vi "fft_kf_update.vi"(9 "Measurement":cdb[](array[numeric]) format="%#_3p", 10 "Measure noise RMS":dbl[](array[numeric]) format="%#_3e", 11 "KF in":T7 {"K" format="%#_2g"; "y lim" format="%#_3g"; "x lim" format="%#_2g"; "P" format="%#_2g"; "H" format="%#_3g"; "x" format="%#_3g"; "Q" format="%#_2g"; "R" format="%#_2g"; "B" format="%#_2g"; "A" format="%#_3g"}) -> (2 "KF out":T7 {"K" format="%#_2g"; "y lim" format="%#_3g"; "x lim" format="%#_2g"; "P" format="%#_2g"; "H" format="%#_3g"; "x" format="%#_3g"; "Q" format="%#_2g"; "R" format="%#_2g"; "B" format="%#_2g"; "A" format="%#_3g"}, 3 "KF estimate":cdb[](array[numeric]) format="%#_3f")   [LabVIEW 2026]
uses:
  utilities/kalman_filter.ctl
  <vilib>/Analysis/Matrix/Datatypes/RealMatrix.ctl
  ilemt_config.ctl
  system/IO_params.ctl
  stft_params.ctl
  <vilib>/Analysis/4window.llb/windowTd.ctl
  filter_params.ctl
  detrend_mode.ctl
  <vilib>/Analysis/Matrix/Numeric/Conversions/Array To Matrix - RA2.vi
  <vilib>/Analysis/Matrix/NI_Matrix.lvlib
  <vilib>/Analysis/NI_AALPro.lvlib
panel:
  in  "Config":T1={"IO params"={"Conversion"={"Rate"=4.0, "Num cards"=2, "Out channels"=4}, "Carriers"={"Phase shift"=180.0, "Levels"=[[0.8, 0.8, 0.8], [0.03, 0.03, 0.03]], "Delay samples"=73.15}, "TCP"={"Host"="192.168.1.15", "Port"=6666, "Buffering"=6, "Timeout"=6}, "Input channel sign"=[1, 1, 1]}, "High rate STFT"={"Win param"=101.5, "Window type"=61, "Win order"=2, "DFT size"=64, "Channels"=[7], "Oversample"=64}, "Low rate STFT"={"Win param"=120.0, "Window type"=61, "Win order"=8, "DFT size"=64, "Channels"=[7], "Oversample"=64}, "Filtering "=[]} {"Filtering"."Distortion"."Limit" format="%#_3p"; "Filtering"."Distortion"."LF cut" format="%#_3p"; "Filtering"."Kalman"."Measure noise" format="%#_3p"; "Filtering"."Kalman"."Process noise" format="%#_3p"; "Filtering"."Hum"."Limit" format="%#_3p"; "Filtering"."Hum"."Frequency" format="%#_4p"; "Low rate STFT"."Oversample" min=1 step=1; "Low rate STFT"."Channels" min=0 step=1; "Low rate STFT"."DFT size" min=1 step=1; "Low rate STFT"."Window type" items=["Rectangle"=0, "Hanning"=1, "Hamming"=2, "Blackman-Harris"=3, "Exact Blackman"=4, "Blackman"=5, "Flat Top"=6, "4 Term B-Harris "=7, "7 Term B-Harris"=8, "Low Sidelobe"=9, "Blackman Nuttall"=11, "Triangle"=30, "Bartlett-Hanning"=31, "Bohman"=32, "Parzen"=33, "Welch"=34, "Kaiser"=60, "Dolph-Chebyshev"=61, "Gaussian"=62]; "High rate STFT"."Oversample" min=1 step=1; "High rate STFT"."Channels" min=0 step=1; "High rate STFT"."DFT size" min=1 step=1; "High rate STFT"."Window type" items=["Rectangle"=0, "Hanning"=1, "Hamming"=2, "Blackman-Harris"=3, "Exact Blackman"=4, "Blackman"=5, "Flat Top"=6, "4 Term B-Harris "=7, "7 Term B-Harris"=8, "Low Sidelobe"=9, "Blackman Nuttall"=11, "Triangle"=30, "Bartlett-Hanning"=31, "Bohman"=32, "Parzen"=33, "Welch"=34, "Kaiser"=60, "Dolph-Chebyshev"=61, "Gaussian"=62]; "IO params"."Input channel sign" min=-1 max=1 step=1; "IO params"."Carriers"."Levels" min=0.0 step=0.1; "IO params"."Conversion"."Rate" format="%#_8g"}
  in  "Current/sensor index":i32 min=0 max=1 step=1
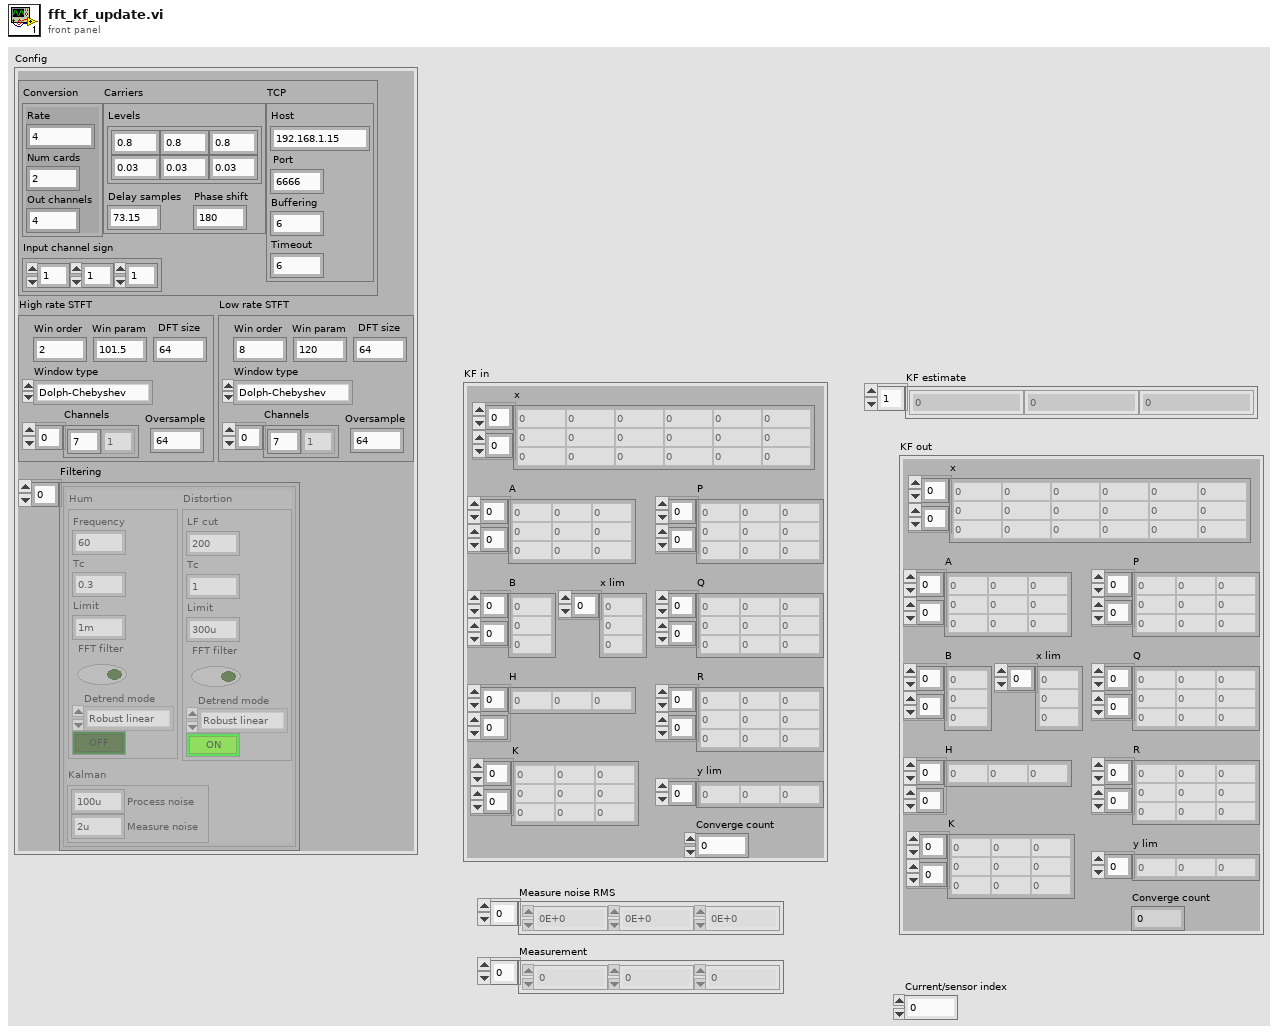
[diagram p1: front panel]
types:
  T1 = typedef "ilemt_config.ctl" = cluster{"IO params":T2, "High rate STFT":T3, "Low rate STFT":T3, "Filtering ":T5[]}
  T2 = typedef "IO_params.ctl" = cluster{"Conversion":cluster{"Rate":dbl, "Num cards":u32, "Out channels":u32}, "Carriers":cluster{"Phase shift":dbl, "Levels":dbl[][], "Delay samples":dbl}, "TCP":cluster{"Host":string, "Port":i32, "Buffering":u32, "Timeout":u32}, "Input channel sign":i32[]}
  T3 = typedef "stft_params.ctl" = cluster{"Win param":dbl, "Window type":T4, "Win order":i32, "DFT size":i32, "Channels":i32[], "Oversample":i32}
  T4 = typedef "NI_AALPro.lvlib/windowTd.ctl" = u32
  T5 = typedef "filter_params.ctl" = cluster{"Hum":cluster{"Frequency":dbl, "Tc":dbl, "Limit":dbl, "FFT filter":bool, "Detrend mode":T6, "Enable":bool}, "Kalman":cluster{"Process noise":dbl, "Measure noise":dbl}, "Distortion":cluster{"LF cut":dbl, "Tc":dbl, "Limit":dbl, "FFT filter":bool, "Detrend mode":T6, "Enable":bool}}
  T6 = typedef "detrend_mode.ctl" = enum16{"Zero mean", "Linear", "Robust linear"}
  T7 = typedef "kalman_filter.ctl" = cluster{"A":T8, "B":T8, "H":T8, "Q":T8, "R":T8, "x":T8, "P":T8, "x lim":dbl[], "y lim":dbl[], "K":T8, "Converge count":i32}
  T8 = typedef "NI_Matrix.lvlib/RealMatrix.ctl" = dbl[][]
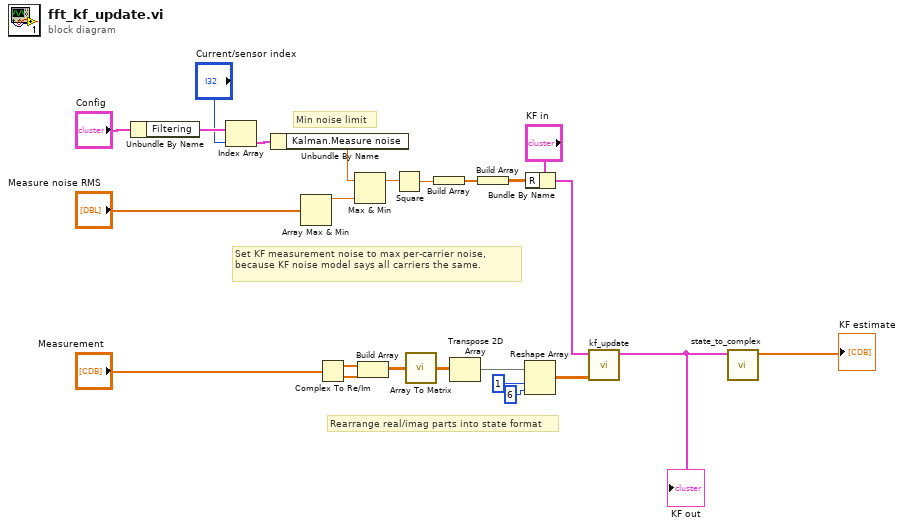
[diagram p0: block diagram]
diagram:
  # "Min noise limit"
  # "Rearrange real/imag parts into state format"
  # "Set KF measurement noise to max per-carrier noise, because KF noise model says all carriers the same."
  n1 = Unbundle By Name("Config") -> ("Filtering"=w9:T5[])
  n2 = Index Array(array=w9, index="Current/sensor index") -> (element=w8:T5)
  n3 = Unbundle By Name(w8) -> ("Kalman.Measure noise"=w3:dbl)
  n4 = Array Max & Min(array="Measure noise RMS") -> (max value=w4:dbl)  [unwired: 3 out]
  n5 = Complex To Re/Im(x + iy="Measurement") -> (x=w12:dbl[], y=w13:dbl[])
  n6 = Max & Min(x=w3, y=w4) -> (max(x,y)=w2:dbl)  [unwired: 1 out]
  n7 = Build Array(w12, w13) -> (w19:dbl[][])
  n8 = Square(x=w2) -> (x^2=w1:dbl)
  n9 = call-poly <vilib>:"Array To Matrix.vi"("Real 2D Array"=w19) -> ("Real Matrix"=w20:T8)
  n10 = Build Array(w1) -> (w15:dbl[])
  n11 = Transpose 2D Array(2D array=w20) -> (transposed array=w18:T8)
  n12 = Build Array(w15) -> (w16:T8)
  n13 = Reshape Array(w18, 1 ("dimension size"), 6 ("dimension size")) -> (w23:T8)
  n14 = Bundle By Name(cluster="KF in", "R"=w16) -> (w17:T7)
  n15 = call "kf_update.vi"("z"=w23, "KF in"=w17) -> ("KF out"=w10:T7)  [unwired: 8 in, 1 out]
  "KF out" <- w10
  n16 = call "state_to_complex.vi"("KF in"=w10) -> ("Amplitudes"=→"KF estimate":cdb[])  [unwired: 10 in]
